vi "UMLEditor ScriptTask.vi"() -> ()   [LabVIEW 2016]
uses:
  <resource>/Framework/Providers/Open_GDS/ClassProviders/Common/CommonVIs/CommonVIs_ClassNamePathType.ctl
  <vilib>/Utility/config.llb/Read Key (String).vi
  <vilib>/Utility/config.llb/Read Key (Path).vi
  <vilib>/Utility/config.llb/Read Key (Boolean).vi
  <vilib>/Utility/config.llb/NI_LVConfig.lvlib
panel:
  in  "Case Constant\n(See Context Help)":bool
  out "error out":errorcluster
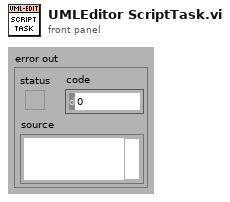
[diagram p1: front panel]
types:
  T1 = cluster{"VIRef":refnum<vi>, "ScripPath":path, "Classes":cluster{"ClassPath":path, "LLB":bool, "Name":string, "SUB":bool, "Attr":string, "BasePath":path, "CompAgg":path[], "CompAggNames":string[]}[], "ObjectRefsToFix":cluster{"classObjectRefPath":path, "Name":string}[], "TemplateRef":refnum<vi>, "Types":cluster{"Name":string, "Path":path, "Attr":string}[], "Queue":refnum<queue>, "WaitForWiz":bool}
  T2 = enum32{"Bad", "Idle", "Run top level", "Running"}
  T3 = cluster{"Name":string, "Path":path, "Attr":string}[]
  T4 = cluster{"ClassPath":path, "LLB":bool, "Name":string, "SUB":bool, "Attr":string, "BasePath":path, "CompAgg":path[], "CompAggNames":string[]}[]
  T5 = cluster{"Name":string, "Path":path, "Attr":string}
  T6 = cluster{"classObjectRefPath":path, "Name":string}[]
  T7 = cluster{"ClassPath":path, "LLB":bool, "Name":string, "SUB":bool, "Attr":string, "BasePath":path, "CompAgg":path[], "CompAggNames":string[]}
  T8 = typedef "NI_LVConfig.lvlib/Config Data RefNum.ctl" = refnum<k1>
  T9 = cluster{"classObjectRefPath":path, "Name":string}
  T10 = typedef "imagedata.ctl" = cluster{"image type":i32, "image depth":i32, "image":u8[], "mask":u8[], "colors":u32[], "Rectangle":cluster{"left":i16, "top":i16, "right":i16, "bottom":i16}}
  T11 = typedef "CommonVIs_ClassNamePathType.ctl" = cluster{"ClassNamn":string, "ClassPath":path, "InterfaceClass":bool}
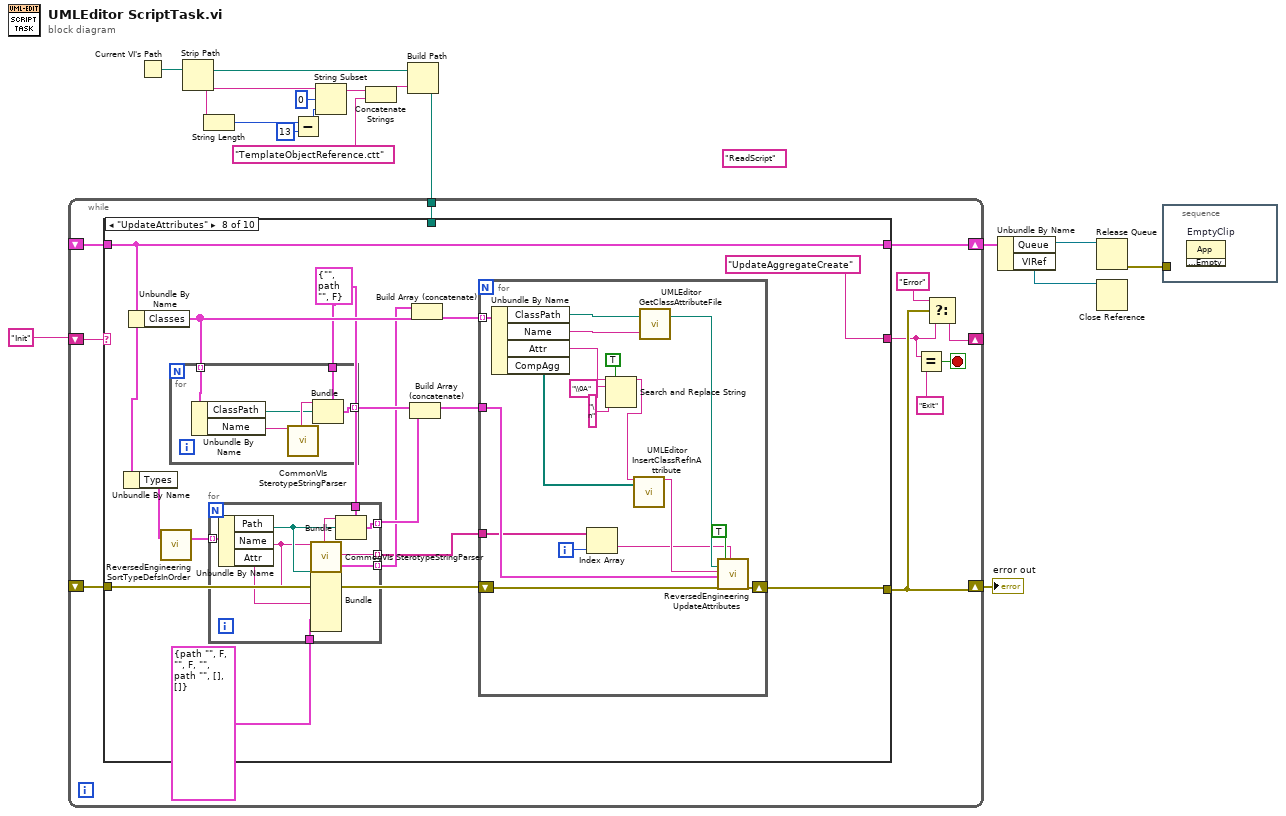
[diagram p0: block diagram]
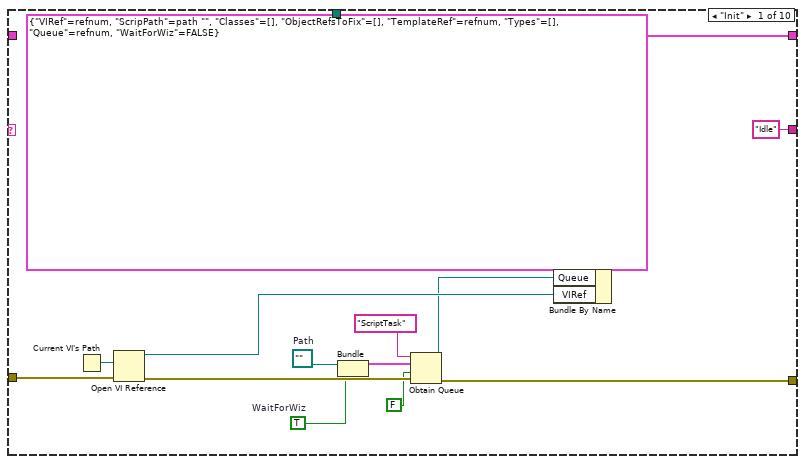
[diagram p2: hidden frame]
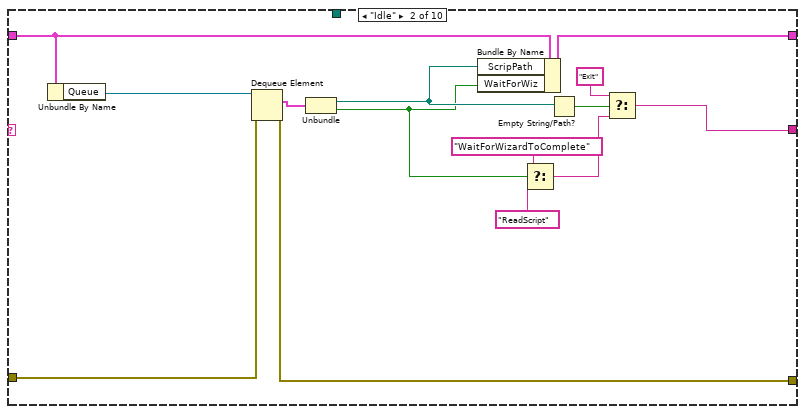
[diagram p3: hidden frame]
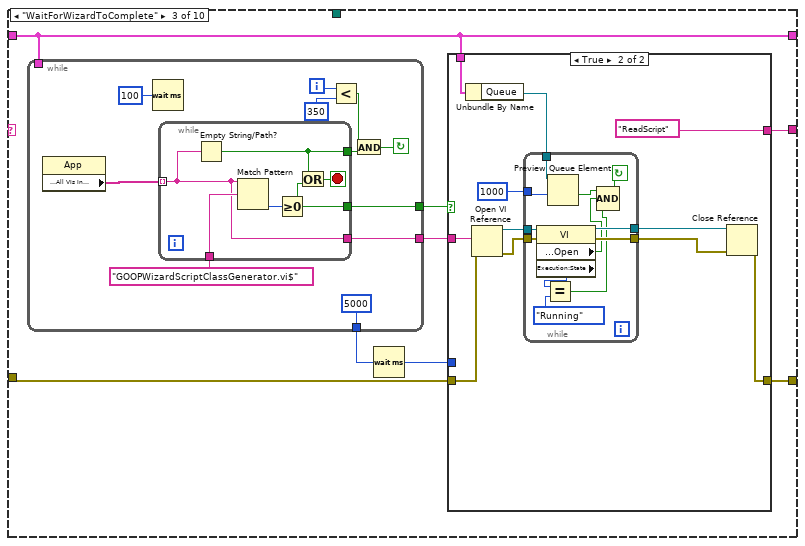
[diagram p4: hidden frame]
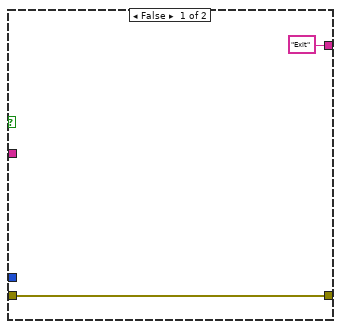
[diagram p5: hidden frame]
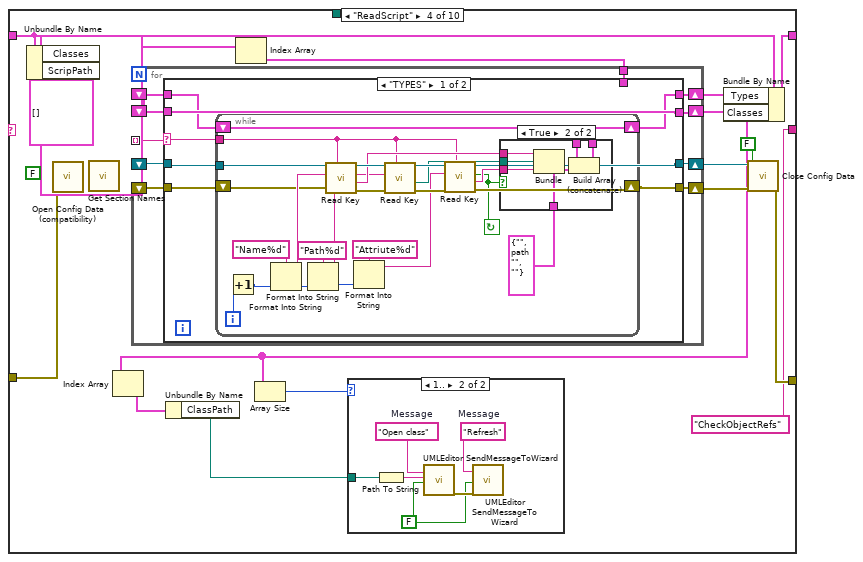
[diagram p6: hidden frame]
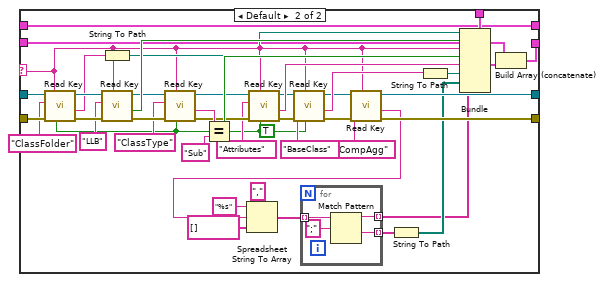
[diagram p9: hidden frame]
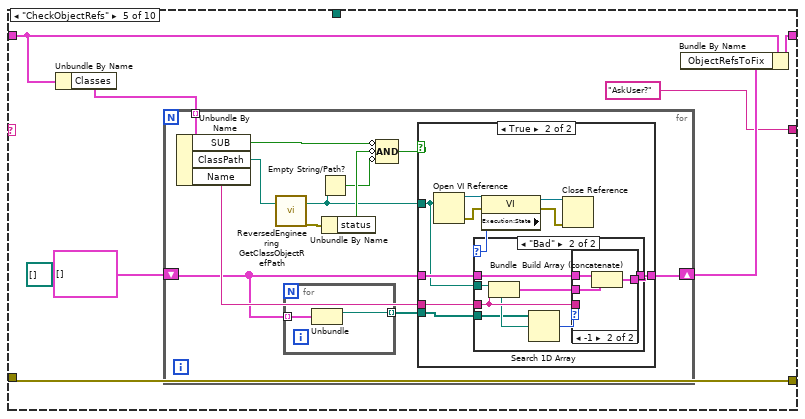
[diagram p10: hidden frame]
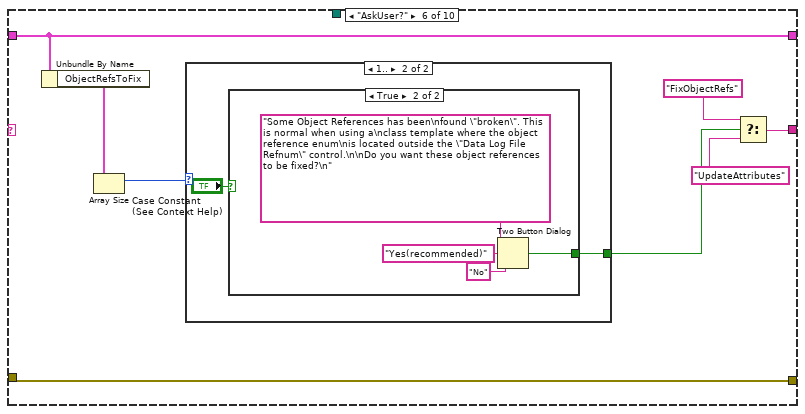
[diagram p14: hidden frame]
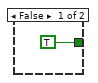
[diagram p16: hidden frame]
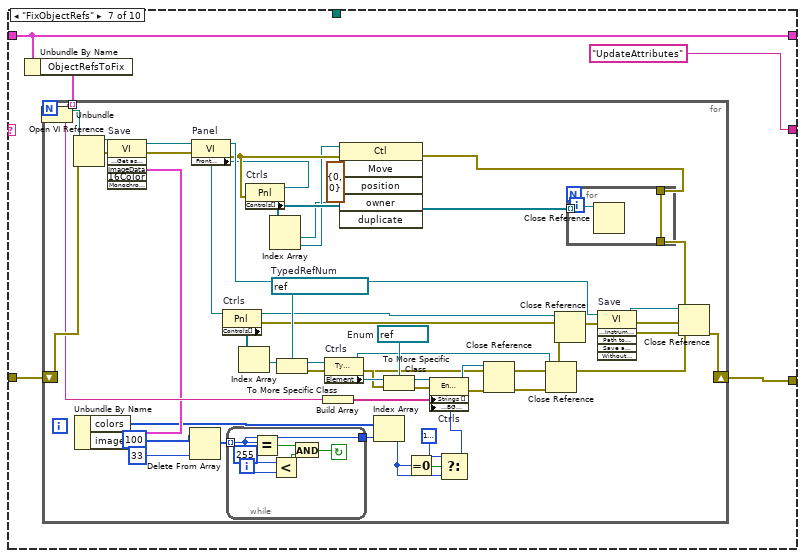
[diagram p17: hidden frame]
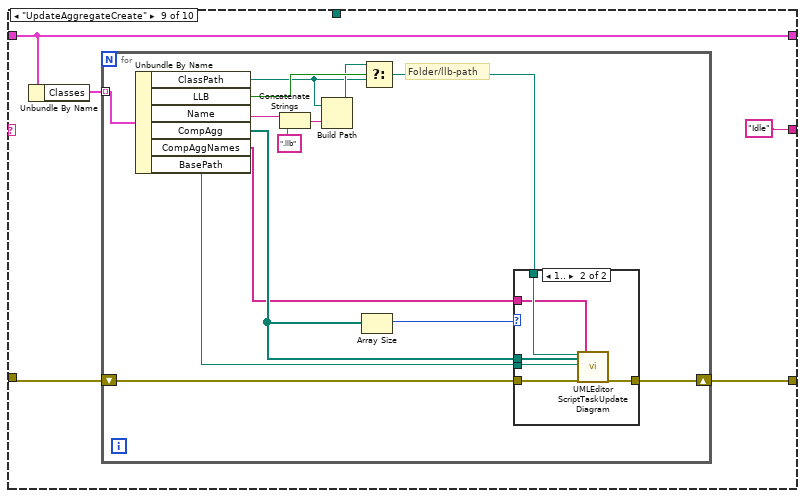
[diagram p18: hidden frame]
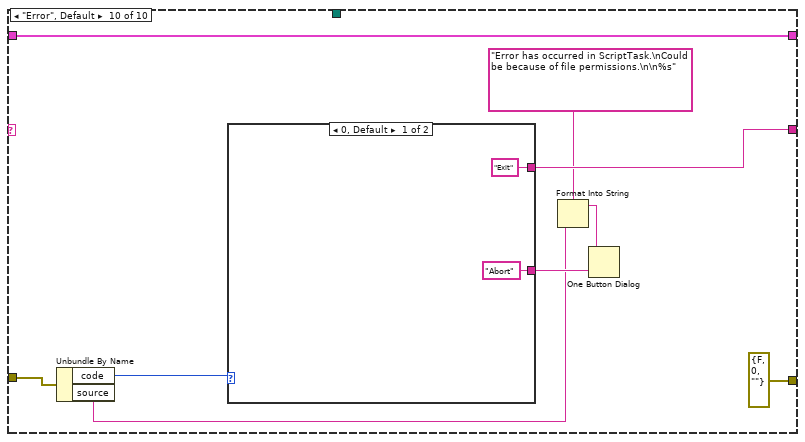
[diagram p20: hidden frame]
diagram:
  (unwired) "ReadScript" ("f")
  n1 = Current VI's Path() -> (path=w12:path)
  n2 = Strip Path(path=w12) -> (stripped path=w6:path, name=w11:string)
  n3 = String Length(string=w11) -> (length=w10:i32)
  n4 = Subtract(x=w10, y=13) -> (x-y=w8:i32)
  n5 = String Subset(string=w11, offset (0)=0, length (rest)=w8) -> (substring=w7:string)
  n6 = Concatenate Strings(w7, "TemplateObjectReference.ctt" ("string")) -> (w5:string)
  n7 = Build Path(base path=w6, name or relative path=w5) -> (appended path=w2:path)
  n8 = while {
    shift-right: [w25] -> _
    shift-left: "Init" -> [w28]
    shift-right: [w26] -> w1
    shift-left: _ -> [w27]
    shift-right: [w20] -> w16
    shift-left: _ -> [w19]
    tunnel: w2 -> [w18]
    stop <- w21 stop-if-true
    n9 = case shown="\"UpdateAttributes\"" w28 {
      tunnel: w27 -> [w38 w55 w61 w123 w234 w278 w293 w367 w403 w434]
      tunnel: [w37 w54 w60 w120 w234 w278 w294 w366 w402 errorcluster {"status"=FALSE, "code"=0, "source"=""} ("error out")] -> w26
      tunnel: ["Idle" w51 w63 "CheckObjectRefs" "AskUser?" ("f") w282 "UpdateAttributes" "UpdateAggregateCreate" "Idle" w432] -> w23
      tunnel: [w34 w49 w59 w118 w237 w277 w295 w364 w405 w436] -> w20
      tunnel: w19 -> [_ w50 w59 w119 w238 w277 w295 w364 w405 w436]
      tunnel: w18 -> [_ _ _ _ _ _ _ _ _ _]
      frame "Init" {
        w32 = path ""  # Path
        w30 = TRUE  # WaitForWiz
        n10 = Current VI's Path() -> (path=w41:path)
        n11 = Open VI Reference(vi path=w41, error in (no error)=w38) -> (vi reference=w35:refnum<vi>, error out=w40:errorcluster)  [unwired: 4 out]
        n12 = Bundle("Path"=w32, "WaitForWiz"=w30) -> (w31:cluster{"Path":path, "WaitForWiz":bool})  [unwired: 1 out]
        n13 = Obtain Queue(name (unnamed)="ScriptTask", element data type=w31, create if not found? (T)=FALSE, error in (no error)=w40) -> (queue out=w29:refnum<queue>, error out=w37:errorcluster)  [unwired: 1 in, 1 out]
        n14 = Bundle By Name(cluster=T1 {"VIRef"=refnum, "ScripPath"=path "", "Classes"=[], "ObjectRefsToFix"=[], "TemplateRef"=refnum, "Types"=[], "Queue"=refnum, "WaitForWiz"=FALSE}, "Queue"=w29, "VIRef"=w35) -> (w34:T1)
      }
      frame "Idle" {
        n15 = Unbundle By Name(w50) -> ("Queue"=w56:refnum<queue>)
        n16 = Dequeue Element(queue=w56, error in (no error)=w55) -> (element=w48:cluster{"Path":path, "WaitForWiz":bool}, error out=w54:errorcluster)  [unwired: 3 out]
        n17 = Unbundle(w48) -> ("Path"=w47:path, "WaitForWiz"=w46:bool)
        n18 = Bundle By Name(cluster=w50, "ScripPath"=w47, "WaitForWiz"=w46) -> (w49:T1)
        n19 = Select(t="WaitForWizardToComplete" ("f"), s=w46, f="ReadScript") -> (s? t:f=w44:string)
        n20 = Empty String/Path?(string/path=w47) -> (empty?=w52:bool)
        n21 = Select(t="Exit", s=w52, f=w44) -> (s? t:f=w51:string)
      }
      frame "WaitForWizardToComplete" {
        n22 = while {
          tunnel: [w93] -> w64
          tunnel: [w92] -> w62
          tunnel: w59 -> [_]
          tunnel: [u32 5000 ("milliseconds to wait")] -> w58
          i -> [w98]
          stop <- w94 continue-if-true
          n23 = property class="App"() -> ("Application:All VIs In Memory"=w100:string[])  [unwired: 2 in, 2 out]
          n24 = Wait (ms)(milliseconds to wait=u32 100) -> ()  [unwired: 1 out]
          n25 = while {
            tunnel: w100 -> [w101] mode=indexing
            tunnel: "GOOPWizardScriptClassGenerator.vi$" -> [w106]
            tunnel: [w103] -> w96
            tunnel: [w102] -> w93
            tunnel: [w101] -> w92
            stop <- w104 stop-if-true
            n26 = Empty String/Path?(string/path=w101) -> (empty?=w103:bool)
            n27 = Match Pattern(string=w101, regular expression=w106) -> (offset past match=w105:i32)  [unwired: 4 out]
            n28 = Greater Or Equal To 0?(x=w105) -> (x >= 0?=w102:bool)
            n29 = Or(x=w103, y=w102) -> (x .or. y?=w104:bool)
          }
          n30 = Less?(x=w98, y=350) -> (x < y?=w95:bool)
          n31 = And(x=w95, y=w96) -> (x .and. y?=w94:bool)
        }
        n32 = Wait (ms)(milliseconds to wait=w58) -> (millisecond timer value=w57:u32)
        n33 = case shown="True" w64 {
          tunnel: ["Exit" "ReadScript" ("f")] -> w63
          tunnel: w62 -> [_ w77]
          tunnel: w61 -> [w66 w72]
          tunnel: [w66 w71] -> w60
          tunnel: w59 -> [_ w69]
          tunnel: w57 -> [_ _]
          frame False {
          }
          frame True {
            n34 = Unbundle By Name(w69) -> ("Queue"=w67:refnum<queue>)
            n35 = Open VI Reference(vi path=w77, error in (no error)=w72) -> (vi reference=w76:refnum<vi>, error out=w75:errorcluster)  [unwired: 4 out]
            n36 = while {
              tunnel: w76 -> [w89]
              tunnel: w75 -> [w88]
              tunnel: [w87] -> w74
              tunnel: [w86] -> w73
              tunnel: 1000 ("timeout in ms (-1)") -> [w85]
              tunnel: w67 -> [w84]
              stop <- w78 continue-if-true
              n37 = property class="VI"(reference=w89, error in=w88) -> (reference out=w87:refnum<vi>, error out=w86:errorcluster, "Front Panel Window:Open"=w80:bool, "Execution:State"=w83:T2)
              n38 = Equal?(x=w83, y=T2."Running") -> (x = y?=w79:bool)
              n39 = Preview Queue Element(queue=w84, timeout in ms (-1)=w85) -> (timed out?=w81:bool)  [unwired: 1 in, 3 out]
              n40 = Compound Arithmetic op=AND(w81, w80, w79) -> (w78:bool)
            }
            n41 = Close Reference(reference=w74, error in (no error)=w73) -> (error out=w71:errorcluster)
          }
        }
      }
      frame "ReadScript" {
        n42 = Unbundle By Name(w119) -> ("Classes"=w117:T4, "ScripPath"=w125:path)
        n43 = call <vilib>:"Open Config Data (compatibility).vi"("error in (no error)"=w123, "create file if necessary (T)"=FALSE ("create file if necessary? (T)"), "configuration file path"=w125) -> ("error out"=w130:errorcluster, "refnum"=w129:T8)  [unwired: 6 in, 1 out]
        n44 = call <vilib>:"Get Section Names.vi"("error in (no error)"=w130, "refnum"=w129) -> ("error out"=w127:errorcluster, "section names"=w126:string[], "refnum out"=w128:T8)  [unwired: 7 out]
        n45 = Index Array(array=w117) -> (element=w116:T7)  [unwired: 1 in]
        n46 = for {
          shift-right: [w142] -> w122
          shift-left: w127 -> [w146]
          shift-right: [w143] -> w121
          shift-left: w128 -> [w145]
          tunnel: w126 -> [w141] mode=indexing
          tunnel: w116 -> [w144]
          shift-right: [w139] -> w108
          shift-left: T4 [] -> [w140]
          shift-right: [w138] -> w110
          shift-left: T3 [] -> [w137]
          n47 = case shown="\"TYPES\"" w141 {
            selector: w141 -> [w153 w189]
            tunnel: w146 -> [w152 w228]
            tunnel: w145 -> [w150 w227]
            tunnel: w144 -> [_ w220]
            tunnel: [w150 w200] -> w143
            tunnel: [w151 w199] -> w142
            tunnel: [w149 w188] -> w139
            tunnel: w140 -> [w149 w187]
            tunnel: w137 -> [w148 w185]
            tunnel: [w147 w185] -> w138
            frame "TYPES" {
              n48 = while {
                tunnel: w150 -> [w175]
                tunnel: w153 -> [w160]
                shift-right: [w157] -> w151
                shift-left: w152 -> [w158]
                shift-right: [w155] -> w147
                shift-left: w148 -> [w156]
                i -> [w170]
                stop <- w154 continue-if-true
                n49 = Increment(x=w170) -> (x+1=w172:i32)
                n50 = Format Into String(format string="Name%d", w172) -> (resulting string=w169:string)  [unwired: 2 in, 1 out]
                n51 = Format Into String(format string="Path%d", w172) -> (resulting string=w165:string)  [unwired: 2 in, 1 out]
                n52 = call-poly <vilib>:"Read Key.vi"("section"=w160, "error in (no error)"=w158, "key"=w169, "refnum"=w175) -> ("error out"=w166:errorcluster, "value"=w168:string, "refnum out"=w167:T8)  [unwired: 2 in, 3 out]
                n53 = Format Into String(format string="Attriute%d", w172) -> (resulting string=w159:string)  [unwired: 2 in, 1 out]
                n54 = call-poly <vilib>:"Read Key.vi"("section"=w160, "error in (no error)"=w166, "key"=w165, "refnum"=w167) -> ("error out"=w161:errorcluster, "value"=w164:path, "refnum out"=w162:T8)  [unwired: 1 in, 4 out]
                n55 = call-poly <vilib>:"Read Key.vi"("section"=w160, "error in (no error)"=w161, "key"=w159, "refnum"=w162) -> ("error out"=w157:errorcluster, "value"=w163:string, "found?"=w154:bool)  [unwired: 2 in, 3 out]
                n56 = case shown="True" w154 {
                  tunnel: T5 {"Name"="", "Path"=path "", "Attr"=""} -> [_ w184]
                  tunnel: w168 -> [_ w182]
                  tunnel: w164 -> [_ w181]
                  tunnel: w163 -> [_ w180]
                  tunnel: w156 -> [w177 w179]
                  tunnel: [w177 w178] -> w155
                  frame False {
                  }
                  frame True {
                    n57 = Bundle(cluster=w184, "Name"=w182, "Path"=w181, "Attr"=w180) -> (w183:T5)
                    n58 = Build Array (concatenate)(w179, w183) -> (w178:T3)
                  }
                }
              }
            }
            frame Default {
              w206 = TRUE ("read raw string? (F)")
              n59 = call-poly <vilib>:"Read Key.vi"("read raw string? (F)"=w206, "section"=w189, "error in (no error)"=w228, "key"="ClassFolder", "refnum"=w227) -> ("error out"=w226:errorcluster, "value"=w222:string, "refnum out"=w225:T8)  [unwired: 1 in, 3 out]
              n60 = String To Path(string=w222) -> (path=w205:path)
              n61 = call-poly <vilib>:"Read Key.vi"("section"=w189, "error in (no error)"=w226, "key"="LLB", "refnum"=w225) -> ("error out"=w218:errorcluster, "value"=w221:bool, "refnum out"=w219:T8)  [unwired: 1 in, 4 out]
              n62 = call-poly <vilib>:"Read Key.vi"("read raw string? (F)"=w206, "section"=w189, "error in (no error)"=w218, "key"="ClassType", "refnum"=w219) -> ("error out"=w212:errorcluster, "value"=w216:string, "refnum out"=w213:T8)  [unwired: 1 in, 3 out]
              n63 = Equal?(x=w216, y="Sub") -> (x = y?=w214:bool)
              n64 = call-poly <vilib>:"Read Key.vi"("read raw string? (F)"=w206, "section"=w189, "error in (no error)"=w212, "key"="Attributes", "refnum"=w213) -> ("error out"=w210:errorcluster, "value"=w209:string, "refnum out"=w207:T8)  [unwired: 1 in, 3 out]
              n65 = call-poly <vilib>:"Read Key.vi"("read raw string? (F)"=w206, "section"=w189, "error in (no error)"=w210, "key"="BaseClass", "refnum"=w207) -> ("error out"=w201:errorcluster, "value"=w203:string, "refnum out"=w202:T8)  [unwired: 1 in, 3 out]
              n66 = call-poly <vilib>:"Read Key.vi"("section"=w189, "error in (no error)"=w201, "key"="CompAgg", "refnum"=w202) -> ("error out"=w199:errorcluster, "value"=w197:string, "refnum out"=w200:T8)  [unwired: 2 in, 3 out]
              n67 = Spreadsheet String To Array(delimiter (Tab)=",", format string="%s", spreadsheet string=w197, array type (2D Dbl)=string[] []) -> (array=w192:string[])
              n68 = for {
                tunnel: w192 -> [w232] mode=indexing
                tunnel: [w230] -> w191 mode=indexing
                tunnel: [w229] -> w190 mode=indexing
                n69 = Match Pattern(string=w232, regular expression=";") -> (before substring=w229:string, after substring=w230:string)  [unwired: 3 out]
              }
              n70 = String To Path(string=w191) -> (path=w193:path[])
              n71 = String To Path(string=w203) -> (path=w204:path)
              n72 = Bundle(cluster=w220, "ClassPath"=w205, "LLB"=w221, "Name"=w189, "SUB"=w214, "Attr"=w209, "BasePath"=w204, "CompAgg"=w193, "CompAggNames"=w190) -> (w186:T7)
              n73 = Build Array (concatenate)(w187, w186) -> (w188:T4)
            }
          }
        }
        n74 = Index Array(array=w108) -> (element=w114:T7)  [unwired: 1 in]
        n75 = Unbundle By Name(w114) -> ("ClassPath"=w113:path)
        n76 = Array Size(array=w108) -> (size(s)=w107:i32)
        n77 = case shown="1.." w107 {
          tunnel: w113 -> [_ w131]
          frame 0, Default {
          }
          frame 1.. {
            w132 = "Refresh"  # Message
            w133 = FALSE ("AllowErrorPopup(True)")
            w136 = "Open class"  # Message
            n78 = Path To String(path=w131) -> (string=w135:string)
            n79 = call <resource>:"UMLEditor SendMessageToWizard.vi"("MessageType"=w136, "MessageData"=w135, "AllowErrorPopup(True)"=w133) -> ("error out"=w134:errorcluster)  [unwired: 1 in, 15 out]
            n80 = call <resource>:"UMLEditor SendMessageToWizard.vi"("MessageType"=w132, "AllowErrorPopup(True)"=w133, "error in (no error)"=w134) -> ()  [unwired: 1 in, 16 out]
          }
        }
        n81 = Bundle By Name(cluster=w119, "Types"=w110, "Classes"=w108) -> (w118:T1)
        n82 = call <vilib>:"Close Config Data.vi"("error in (no error)"=w122, "write file if changed (T)"=FALSE ("write configuration file? (T)"), "refnum"=w121) -> ("error out"=w120:errorcluster)  [unwired: 8 out]
      }
      frame "CheckObjectRefs" {
        (unwired) path[] []
        n83 = Unbundle By Name(w238) -> ("Classes"=w239:T4)
        n84 = for {
          tunnel: w239 -> [w251] mode=indexing
          shift-right: [w244] -> w236
          shift-left: T6 [] -> [w242]
          n85 = Unbundle By Name(w251) -> ("SUB"=w240:bool, "ClassPath"=w250:path, "Name"=w243:string)
          n86 = call <resource>:"ReversedEngineering GetClassObjectRefPath.vi"("llbClassPath"=w250) -> ("classObjectRefPath"=w245:path, "error out"=w249:errorcluster)  [unwired: 1 in, 16 out]
          n87 = for {
            tunnel: w242 -> [w253] mode=indexing
            tunnel: [w252] -> w241 mode=indexing
            n88 = Unbundle(w253) -> ("classObjectRefPath"=w252:path)  [unwired: 1 out]
          }
          n89 = Empty String/Path?(string/path=w245) -> (empty?=w246:bool)
          n90 = Unbundle By Name(w249) -> ("status"=w247:bool)
          n91 = Compound Arithmetic op=AND(invert w240, invert w247, invert w246) -> (w248:bool)
          n92 = case shown="True" w248 {
            tunnel: w245 -> [_ w256]
            tunnel: w242 -> [w254 w259]
            tunnel: [w254 w258] -> w244
            tunnel: w243 -> [_ w257]
            tunnel: w241 -> [_ w255]
            frame False {
            }
            frame True {
              n93 = Open VI Reference(vi path=w256) -> (vi reference=w264:refnum<vi>, error out=w263:errorcluster)  [unwired: 2 in, 3 out]
              n94 = property class="VI"(reference=w264, error in=w263) -> (reference out=w262:refnum<vi>, error out=w261:errorcluster, "Execution:State"=w260:T2)
              n95 = case shown="\"Bad\"" w260 {
                tunnel: w259 -> [w265 w269]
                tunnel: [w265 w272] -> w258
                tunnel: w257 -> [_ w270]
                tunnel: w256 -> [_ w267]
                tunnel: w255 -> [_ w266]
                frame Default {
                }
                frame "Bad" {
                  n96 = Bundle("classObjectRefPath"=w267, "Name"=w270) -> (w268:T9)  [unwired: 1 out]
                  n97 = Search 1D Array(1D array=w266, element=w267) -> (index of element=w271:i32)  [unwired: 1 out]
                  n98 = case shown="-1" w271 {
                    tunnel: w269 -> [w273 w276]
                    tunnel: [w273 w275] -> w272
                    tunnel: w270 -> [_ _]
                    tunnel: w268 -> [_ w274]
                    frame 0, Default {
                    }
                    frame -1 {
                      n99 = Build Array (concatenate)(w276, w274) -> (w275:T6)
                    }
                  }
                }
              }
              n100 = Close Reference(reference=w262, error in (no error)=w261) -> ()  [unwired: 1 out]
            }
          }
        }
        n101 = Bundle By Name(cluster=w238, "ObjectRefsToFix"=w236) -> (w237:T1)
      }
      frame "AskUser?" {
        n102 = Unbundle By Name(w277) -> ("ObjectRefsToFix"=w284:T6)
        n103 = Array Size(array=w284) -> (size(s)=w283:i32)
        n104 = case shown="1.." w283 {
          tunnel: [_ w286] -> w281
          frame 0, Default {
          }
          frame 1.. {
            n105 = case shown="True" "Case Constant\n(See Context Help)" {
              tunnel: [TRUE ("T button?") w288] -> w286
              frame False {
              }
              frame True {
                n106 = Two Button Dialog(message="Some Object References has been\nfound \"broken\". This is normal when using a\nclass template where the object reference enum\nis located outside the \"Data Log File Refnum\" control.\n\nDo you want these object references to be fixed?\n", 1:"No" ("F button name (\"Cancel\")"), 2:"Yes(recommended)" ("T button name (\"OK\")")) -> (T button?=w288:bool)
              }
            }
          }
        }
        n107 = Select(t="FixObjectRefs", s=w281, f="UpdateAttributes") -> (s? t:f=w282:string)
      }
      frame "FixObjectRefs" {
        n108 = Unbundle By Name(w295) -> ("ObjectRefsToFix"=w296:T6)
        n109 = for {
          tunnel: w296 -> [w335] mode=indexing
          shift-right: [w319] -> w294
          shift-left: w293 -> [w343]
          w337 = refnum<vi> refnum  # Enum
          w340 = refnum<vi> refnum  # TypedRefNum
          n110 = Unbundle(w335) -> ("classObjectRefPath"=w334:path, "Name"=w333:string)
          n111 = Open VI Reference(vi path=w334, error in (no error)=w343) -> (vi reference=w311:refnum<vi>, error out=w310:errorcluster)  [unwired: 1 in, 3 out]
          n112 = invoke on="Save" class="VI" method="VI Icon.Get as Image Data"(reference=w311, error in=w310) -> (reference out=w309:refnum<vi>, error out=w308:errorcluster, "ImageData"=w307:T10)  [unwired: 4 in, 3 out]
          n113 = Unbundle By Name(w307) -> ("colors"=w302:u32[], "image"=w306:u8[])
          n114 = Delete From Array(array=w306, length=100, index=33) -> (deleted portion=w305:u8[])  [unwired: 1 out]
          n115 = property on="Panel" class="VI"(reference=w309, error in=w308) -> (reference out=w323:refnum<vi>, error out=w318:errorcluster, "Front Panel"=w312:refnum<vi>)
          n116 = while {
            tunnel: w305 -> [w345] mode=indexing
            tunnel: [w345] -> w303
            i -> [w349]
            stop <- w346 continue-if-true
            w348 = 255
            n117 = Equal?(x=w345, y=w348) -> (x = y?=w350:bool)
            n118 = Less?(x=w349, y=w348) -> (x < y?=w347:bool)
            n119 = And(x=w350, y=w347) -> (x .and. y?=w346:bool)
          }
          n120 = property on="Ctrls" class="Pnl"(reference=w312, error in=w318) -> ("Controls[]"=w344:refnum<vi>[])  [unwired: 2 out]
          n121 = Index Array(array=w344) -> (element #1=w316:refnum<vi>, element #2=w317:refnum<vi>)  [unwired: 2 in]
          n122 = Build Array(w333) -> (w332:string[])
          n123 = invoke class="Ctl" method="Move"(reference=w317, error in=w318, "position"=cluster{"Left":i32, "Top":i32} {"Left"=0, "Top"=0}, "owner"=w316) -> (error out=w314:errorcluster)  [unwired: 2 in, 5 out]
          n124 = Index Array(array=w302, index=w303) -> (element=w299:u32)
          n125 = Equal To 0?(x=w299) -> (x = 0?=w300:bool)
          n126 = Select(t=u32 16777216, s=w300, f=w299) -> (s? t:f=w298:u32)
          n127 = for {
            tunnel: w344 -> [w352] mode=indexing
            tunnel: [w351] -> w313
            tunnel: w314 -> [w351]
            n128 = Close Reference(reference=w352) -> ()  [unwired: 1 in, 1 out]
          }
          n129 = property on="Ctrls" class="Pnl"(reference=w312, error in=w313) -> ("Controls[]"=w342:refnum<vi>[])  [unwired: 2 out]
          n130 = Index Array(array=w342) -> (element=w341:refnum<vi>)  [unwired: 1 in]
          n131 = To More Specific Class(target class=w340, reference=w341, error in=w313) -> (specific class reference=w339:refnum<vi>, error out=w331:errorcluster)
          n132 = property on="Ctrls" class="TypRef"(reference=w339, error in=w331) -> (reference out=w325:refnum<vi>, error out=w330:errorcluster, "Element"=w338:refnum<vi>)
          n133 = To More Specific Class(target class=w337, reference=w338, error in=w330) -> (specific class reference=w336:refnum<vi>, error out=w329:errorcluster)
          n134 = property on="Ctrls" class="Enum"(reference=w336, error in=w329, "Strings []"=w332, "Named Numeric Colors:BG Color"=w298) -> (reference out=w328:refnum<vi>, error out=w327:errorcluster)
          n135 = Close Reference(reference=w328, error in (no error)=w327) -> (error out=w326:errorcluster)
          n136 = Close Reference(reference=w325, error in (no error)=w326) -> (error out=w324:errorcluster)
          n137 = Close Reference(reference=w312, error in (no error)=w324) -> (error out=w322:errorcluster)
          n138 = invoke on="Save" class="VI" method="Save.Instrument"(reference=w323, error in=w322) -> (reference out=w321:refnum<vi>, error out=w320:errorcluster)  [unwired: 4 in, 4 out]
          n139 = Close Reference(reference=w321, error in (no error)=w320) -> (error out=w319:errorcluster)
        }
      }
      frame "UpdateAttributes" {
        w353 = T11 {"ClassNamn"="", "ClassPath"=path "", "InterfaceClass"=FALSE} ("Cluster")
        n140 = Unbundle By Name(w364) -> ("Types"=w356:T3)
        n141 = Unbundle By Name(w364) -> ("Classes"=w360:T4)
        n142 = call <resource>:"ReversedEngineering SortTypeDefsInOrder.vi"("Types"=w356) -> ("TypesOut"=w355:T3)  [unwired: 18 out]
        n143 = for {
          tunnel: w360 -> [w382] mode=indexing
          tunnel: [w379] -> w363 mode=indexing
          tunnel: w353 -> [w378]
          n144 = Unbundle By Name(w382) -> ("ClassPath"=w381:path, "Name"=w380:string)
          n145 = call <resource>:"CommonVIs SterotypeStringParser.vi"("SterotypeStringIn"=w380) -> ("Name"=w383:string)  [unwired: 18 out]
          n146 = Bundle(cluster=w378, "ClassNamn"=w383, "ClassPath"=w381) -> (w379:T11)  [unwired: 1 out]
        }
        n147 = for {
          tunnel: w355 -> [w376] mode=indexing
          tunnel: [w375] -> w361 mode=indexing
          tunnel: T7 {"ClassPath"=path "", "LLB"=FALSE, "Name"="", "SUB"=FALSE, "Attr"="", "BasePath"=path "", "CompAgg"=[], "CompAggNames"=[]} ("input cluster") -> [w374]
          tunnel: [w370] -> w357 mode=indexing
          tunnel: [w369] -> w354 mode=indexing
          tunnel: w353 -> [w368]
          n148 = Unbundle By Name(w376) -> ("Path"=w373:path, "Name"=w372:string, "Attr"=w371:string)
          n149 = call <resource>:"CommonVIs SterotypeStringParser.vi"("SterotypeStringIn"=w372) -> ("Name"=w377:string, "Sterotype"=w369:string)  [unwired: 17 out]
          n150 = Bundle(cluster=w374, "ClassPath"=w373, "Name"=w372, "Attr"=w371) -> (w370:T7)  [unwired: 5 out]
          n151 = Bundle(cluster=w368, "ClassNamn"=w377, "ClassPath"=w373) -> (w375:T11)  [unwired: 1 out]
        }
        n152 = Build Array (concatenate)(w363, w361) -> (w362:T11[])
        n153 = Build Array (concatenate)(w357, w360) -> (w359:T4)
        n154 = for {
          tunnel: w359 -> [w401] mode=indexing
          shift-right: [w399] -> w366
          shift-left: w367 -> [w400]
          tunnel: w362 -> [w394]
          tunnel: w354 -> [w386]
          i -> [w385]
          n155 = Unbundle By Name(w401) -> ("ClassPath"=w397:path, "Name"=w396:string, "Attr"=w390:string, "CompAgg"=w389:path[])
          n156 = Index Array(array=w386, index=w385) -> (element=w384:string)
          n157 = Search and Replace String(replace all?=TRUE ("replace all? (F)"), input string=w390, search string="\\0A", replace string="\n" ("replace string (\"\")")) -> (result string=w388:string)  [unwired: 1 in, 6 out]
          n158 = call <resource>:"UMLEditor InsertClassRefInAttribute.vi"("AttributeIn"=w388, "CompAgg"=w389) -> ("AttributeOut"=w387:string)  [unwired: 1 in, 16 out]
          n159 = call <resource>:"UMLEditor GetClassAttributeFile.vi"("ClassName"=w396, "ClassPath"=w397) -> ("AttributePath"=w395:path)  [unwired: 1 out]
          n160 = call <resource>:"ReversedEngineering UpdateAttributes.vi"("ClassPath/LvClassRef"=w395, "NewAttributes"=w387, "ClassInfo"=w394, "error in (no error)"=w400, "Don't Prompt (False)"=TRUE, "Stereotype"=w384) -> ("error out"=w399:errorcluster)  [unwired: 13 out]
        }
      }
      frame "UpdateAggregateCreate" {
        n161 = Unbundle By Name(w405) -> ("Classes"=w404:T4)
        n162 = for {
          tunnel: w404 -> [w420] mode=indexing
          shift-right: [w412] -> w402
          shift-left: w403 -> [w413]
          # "Folder/llb-path"
          n163 = Unbundle By Name(w420) -> ("ClassPath"=w414:path, "LLB"=w416:bool, "Name"=w419:string, "CompAgg"=w409:path[], "CompAggNames"=w407:string[], "BasePath"=w410:path)
          n164 = Concatenate Strings(w419, ".llb" ("string")) -> (w417:string)
          n165 = Build Path(base path=w414, name or relative path=w417) -> (appended path=w415:path)
          n166 = Array Size(array=w409) -> (size(s)=w408:i32)
          n167 = Select(t=w415, s=w416, f=w414) -> (s? t:f=w411:path)
          n168 = case shown="1.." w408 {
            tunnel: w413 -> [w421 w427]
            tunnel: [w421 w426] -> w412
            tunnel: w411 -> [_ w425]
            tunnel: w410 -> [_ w424]
            tunnel: w409 -> [_ w423]
            tunnel: w407 -> [_ w422]
            frame 0, Default {
            }
            frame 1.. {
              n169 = call <resource>:"UMLEditor ScriptTaskUpdateDiagram.vi"("Folder/LLB-Path"=w425, "AggregateClassPaths"=w423, "BaseClass Folder/LLB-Path"=w424, "error in (no error)"=w427, "AggregateClassNames"=w422) -> ("error out"=w426:errorcluster)  [unwired: 14 out]
            }
          }
        }
      }
      frame "Error", Default {
        n170 = Unbundle By Name(w434) -> ("code"=w433:i32, "source"=w428:string)
        n171 = case shown="0, Default" w433 {
          tunnel: ["Exit" "Idle"] -> w432
          tunnel: ["Abort" ("button name (\"OK\")") "Continue" ("button name (\"OK\")")] -> w431
          frame 0, Default {
          }
          frame 2..8 {
          }
        }
        n172 = Format Into String(format string="Error has occurred in ScriptTask.\nCould be because of file permissions.\n\n%s" ("message"), w428) -> (resulting string=w429:string)  [unwired: 2 in, 1 out]
        n173 = One Button Dialog(message=w429, button name ("OK")=w431) -> ()  [unwired: 1 out]
      }
    }
    n174 = Equal?(x=w23, y="Exit") -> (x = y?=w21:bool)
    n175 = Select(t="Error", s=w26, f=w23) -> (s? t:f=w25:string)
  }
  "error out" <- w1
  n176 = Unbundle By Name(w16) -> ("Queue"=w15:refnum<queue>, "VIRef"=w14:refnum<vi>)
  n177 = Release Queue(queue=w15) -> (error out=w13:errorcluster)  [unwired: 1 in, 3 out]
  n178 = Close Reference(reference=w14) -> ()  [unwired: 1 in, 1 out]
  n179 = stacked-sequence {
    tunnel: w13 -> [_]
    frame #0 {
      n180 = invoke on="EmptyClip" class="App" method="Clipboard.Empty"() -> ()  [unwired: 3 in, 3 out]
    }
  }
